vi "Test B.vi"(8 "error in (no error)":errorcluster) -> (0 "error out":errorcluster)   [LabVIEW 2019, in "Simple Example(Station1).lvlib"]
uses:
  Simple Example(Station1).lvlib
  400e6fd7-5c57-4563-98c8-4c487ac03ebd.vi
  d135eecd-02d8-4d26-94c7-1196041114e8.vi
  Read Limit(Double Float Array).vi
  LVUT Global 1.vi
  <vilib>/Utility/Data Type/Get Type Information.vi
  <vilib>/Utility/error.llb/Trim Whitespace.vi
  Almost Equal.vi
  Unit Test Engine Tools.lvlib
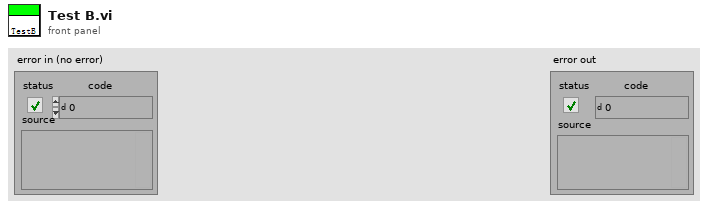
[diagram p1: front panel]
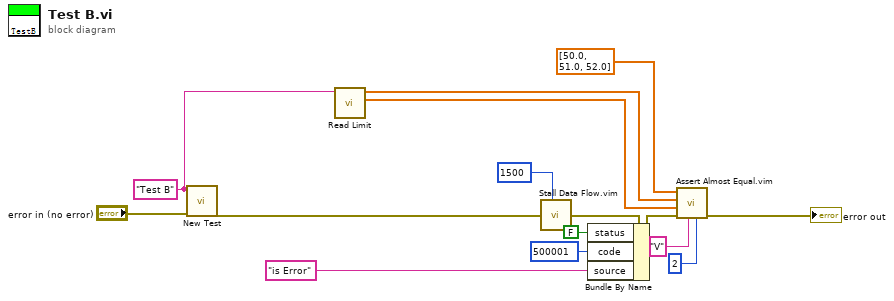
[diagram p0: block diagram]
diagram:
  w3 = "Test B" ("Test")
  n1 = call "New Test.vi"("error in (no error)"="error in (no error)", "Test"=w3) -> ("error out"=w14:errorcluster)  [unwired: 9 in]
  n2 = call-poly "Read Limit.vi"("Test"=w3) -> ("a"=w1:dbl[], "b"=w2:dbl[])  [unwired: 8 in, 1 out]
  n3 = call "Stall Data Flow.vim"("value in"=w14, "milliseconds to wait"=u32 1500) -> ("value out"=w11:errorcluster)  [unwired: 1 out]
  n4 = Bundle By Name(cluster=w11, "status"=FALSE, "code"=500001, "source"="is Error") -> (w8:errorcluster)
  n5 = call "Assert Almost Equal.vim"("precision (2)"=i16 2 ("precision (6)"), "Unit"="V", "error in (no error)"=w8, "a"=w1, "b"=w2, "x"=dbl[] [50.0, 51.0, 52.0]) -> ("error out"=→"error out":errorcluster)  [unwired: 5 in]
